vi "Destroy.vi"(8 "error in":errorcluster, 11 "Sorted Object Dictionary in":refnum<class "Sorted Object Dictionary.lvclass">) -> (0 "error out":errorcluster, 3 "Sorted Object Dictionary out":refnum<class "Sorted Object Dictionary.lvclass">)   [LabVIEW 2020, in "Electronic Datasheet.lvlib" / "Sorted Object Dictionary.lvclass"]
uses:
  Sorted Object Dictionary.lvclass
  Sorted Object Dictionary.lvclass/Sorted Object Dictionary.ctl
  OD Entry/OD Entry.lvclass
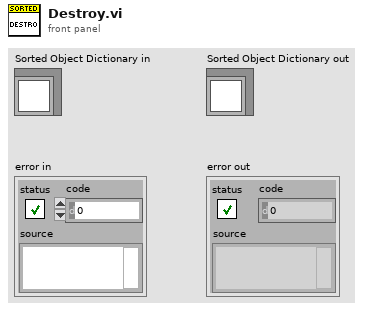
[diagram p1: front panel]
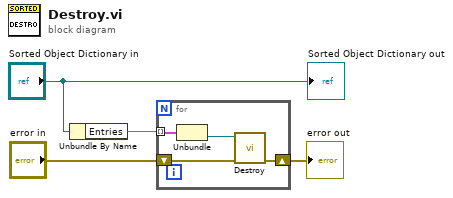
[diagram p0: block diagram]
diagram:
  n1 = Unbundle By Name("Sorted Object Dictionary in") -> ("Entries"=w3:map{u16, refnum<class "OD Entry.lvclass">})
  n2 = for {
    tunnel: w3 -> [w8] mode=indexing
    shift-right: [w5] -> w1
    shift-left: "error in" -> [w6]
    n3 = Unbundle(w8) -> ("OD Entry"=w7:refnum<class "OD Entry.lvclass">)  [unwired: 1 out]
    n4 = call-dynamic "Destroy.vi"("Error In"=w6, "reference in"=w7) -> ("Error Out"=w5:errorcluster)  [unwired: 8 in, 1 out]
  }
  "error out" <- w1
  "Sorted Object Dictionary out" <- "Sorted Object Dictionary in"
